vi "ArduinoLabVIEW.vi"() -> ()   [LabVIEW 2020]
uses:
  <vilib>/httpClient/POSTBuffer.vi
  <vilib>/httpClient/LabVIEWHTTPClient.lvlib
panel:
  out "body":string
  out "headers":string
  out "body 2":string
  out "headers 2":string
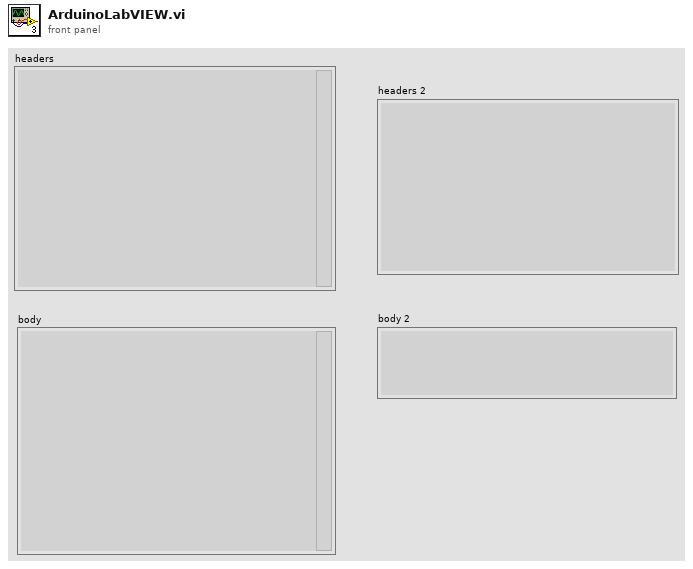
[diagram p1: front panel]
types:
  T1 = cluster{"access_token":string, "token_type":string, "expires_in":i32}
  T2 = typedef "LabVIEWHTTPClient.lvlib/ClientHandle.ctl" = refnum<k1>
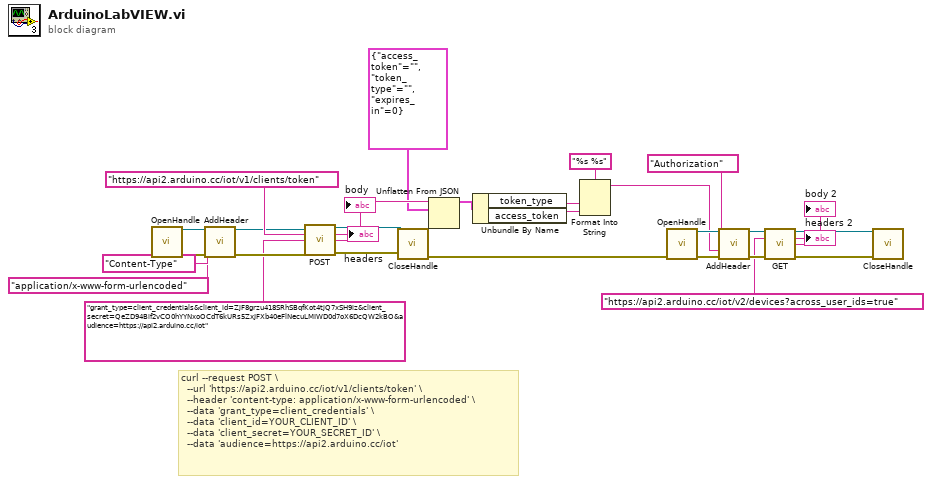
[diagram p0: block diagram]
diagram:
  # "curl --request POST \\\n  --url 'https://api2.arduino.cc/iot/v1/clients/token' \\\n  --header 'content-type: application/x-www-form-urlencoded' \\\n  --data 'grant_type=client_credentials' \\\n  --data 'client_id=YOUR_CLIENT_ID' \\\n  --data 'client_secret=YOUR_SECRET_ID' \\\n  --data 'audience=https://api2.arduino.cc/iot'"
  n1 = call <vilib>:"OpenHandle.vi"() -> ("client handle out"=w29:T2, "error out"=w28:errorcluster)  [unwired: 14 in]
  n2 = call <vilib>:"AddHeader.vi"("client handle"=w29, "header"="Content-Type", "value"="application/x-www-form-urlencoded", "error in (no error)"=w28) -> ("client handle out"=w21:T2, "error out"=w27:errorcluster)  [unwired: 10 in]
  n3 = call-poly <vilib>:"POST.vi"("client handle"=w21, "url"="https://api2.arduino.cc/iot/v1/clients/token", "buffer"="grant_type=client_credentials&client_id=ZjF8grzu418SRhSBqfKot4tjQ7xSH9iz&client_secret=QeZD94Bif2vCO0hYYNxoOCdT6kURs5ZxJFXb40eFlNecuLMIWD0d7oX6DcQW2kBO&audience=https://api2.arduino.cc/iot", "error in (no error)"=w27) -> ("client handle out"=w9:T2, "headers"=→"headers":string, "body"=w20:string, "error out"=w8:errorcluster)  [unwired: 8 in]
  "body" <- w20
  n4 = call <vilib>:"CloseHandle.vi"("client handle"=w9, "error in (no error)"=w8) -> ("error out"=w7:errorcluster)  [unwired: 13 in]
  n5 = Unflatten From JSON(JSON string=w20, type and defaults=T1 {"access_token"="", "token_type"="", "expires_in"=0}) -> (value=w18:T1)  [unwired: 5 in, 1 out]
  n6 = Unbundle By Name(w18) -> ("token_type"=w4:string, "access_token"=w5:string)
  n7 = Format Into String(format string="%s %s", w4, w5) -> (resulting string=w3:string)  [unwired: 2 in, 1 out]
  n8 = call <vilib>:"OpenHandle.vi"("error in (no error)"=w7) -> ("client handle out"=w17:T2, "error out"=w16:errorcluster)  [unwired: 13 in]
  n9 = call <vilib>:"AddHeader.vi"("client handle"=w17, "header"="Authorization", "value"=w3, "error in (no error)"=w16) -> ("client handle out"=w14:T2, "error out"=w13:errorcluster)  [unwired: 10 in]
  n10 = call <vilib>:"GET.vi"("client handle"=w14, "url"="https://api2.arduino.cc/iot/v2/devices?across_user_ids=true", "error in (no error)"=w13) -> ("client handle out"=w2:T2, "headers"=→"headers 2":string, "body"=→"body 2":string, "error out"=w1:errorcluster)  [unwired: 9 in]
  n11 = call <vilib>:"CloseHandle.vi"("client handle"=w2, "error in (no error)"=w1) -> ()  [unwired: 13 in, 1 out]
